vi "mxwScript_API_XMLMakeTargetRefText.vi"(6 "relativeToExistData":T1, 8 "templateData":T5={"tag"="", "index"=-1, "targetRefTemplateType"=enum."OutputAverage", "referencePosition"=enum."Right", "terminalData"={"name"="", "termIsTag"=FALSE, "referencePosition"=enum."TopLeft"}}, 9 "absoluteData":T4, 10 "terminalData":T3, 11 "targetRefType":T2) -> (3 "targetRefText":string)   [LabVIEW 2020]
uses:
  codeGenAPISupport.llb/cgAPI_mxwScript_DrpTmplt_TargetRefTemplateData.ctl
  codeGenAPISupport.llb/cgAPI_mxwScript_DrpTmplt_TargetRefTemplateType.ctl
  codeGenAPISupport.llb/cgAPI_mxwScript_DrpTmplt_ReferencePosition.ctl
  codeGenAPISupport.llb/cgAPI_mxwScript_DrpTmplt_TerminalData.ctl
  codeGenAPISupport.llb/cgAPI_mxwScript_DrpTmplt_AbsoluteData.ctl
  codeGenAPISupport.llb/cgAPI_mxwScript_DrpTmplt_TargetRefType.ctl
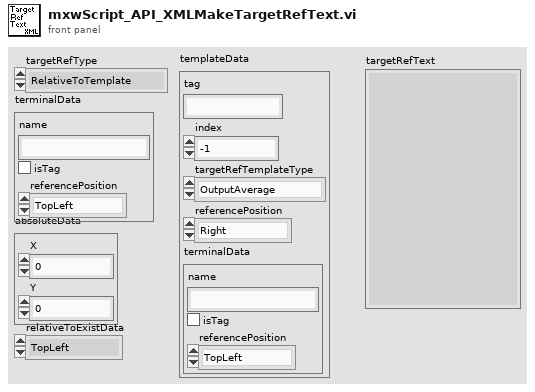
[diagram p1: front panel]
types:
  T1 = typedef "cgAPI_mxwScript_DrpTmplt_ReferencePosition.ctl" = enum16{"TopLeft", "Top", "TopRight", "Left", "Middle", "Right", "BottomLeft", "Bottom", "BottomRight"}
  T2 = typedef "cgAPI_mxwScript_DrpTmplt_TargetRefType.ctl" = enum16{"RelativeToTemplate", "RelativeToTerminal", "AbsoluteOnRoot", "AbsoluteOnTarget", "RelativeToExistOnRoot"}
  T3 = typedef "cgAPI_mxwScript_DrpTmplt_TerminalData.ctl" = cluster{"name":string, "termIsTag":bool, "referencePosition":T1}
  T4 = typedef "cgAPI_mxwScript_DrpTmplt_AbsoluteData.ctl" = cluster{"X":i32, "Y":i32}
  T5 = typedef "cgAPI_mxwScript_DrpTmplt_TargetRefTemplateData.ctl" = cluster{"tag":string, "index":i32, "targetRefTemplateType":T6, "referencePosition":T1, "terminalData":T3}
  T6 = typedef "cgAPI_mxwScript_DrpTmplt_TargetRefTemplateType.ctl" = enum16{"OutputAverage", "Absolute", "Terminal"}
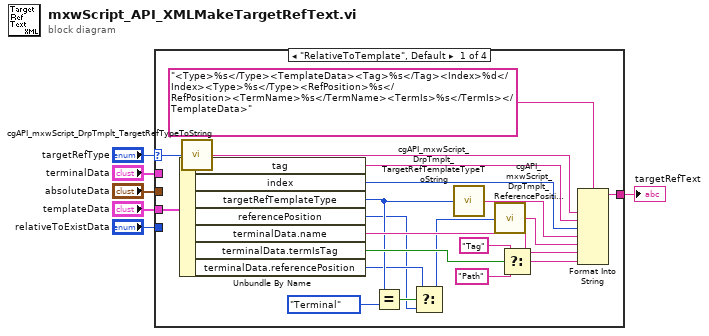
[diagram p0: block diagram]
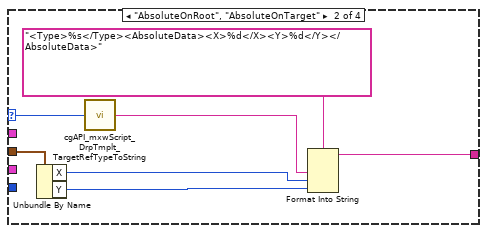
[diagram p2: hidden frame]
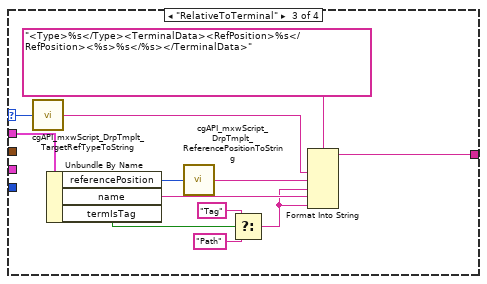
[diagram p3: hidden frame]
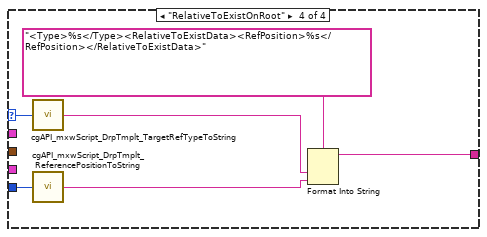
[diagram p4: hidden frame]
diagram:
  n1 = case shown="\"RelativeToTemplate\", Default" "targetRefType" {
    selector: "targetRefType" -> [w13 w28 w37 w49]
    tunnel: "terminalData" -> [_ _ w39 _]
    tunnel: "absoluteData" -> [_ w31 _ _]
    tunnel: "templateData" -> [w26 _ _ _]
    tunnel: [w15 w32 w40 w50] -> w6
    tunnel: "relativeToExistData" -> [_ _ _ w47]
    frame "RelativeToTemplate", Default {
      n2 = Unbundle By Name(w26) -> ("tag"=w24:string, "index"=w23:i32, "targetRefTemplateType"=w12:T6, "referencePosition"=w8:T1, "terminalData.name"=w20:string, "terminalData.termIsTag"=w19:bool, "terminalData.referencePosition"=w9:T1)
      n3 = call "cgAPI_mxwScript_DrpTmplt_TargetRefTypeToString.vi"("targetRefType"=w13) -> ("string"=w14:string)  [unwired: 4 out]
      n4 = Equal?(x=w12, y=cgAPI_mxwScript_DrpTmplt_TargetRefTemplateType."Terminal") -> (x = y?=w10:bool)
      n5 = Select(t=w9, s=w10, f=w8) -> (s? t:f=w7:T1)
      n6 = call "cgAPI_mxwScript_DrpTmplt_TargetRefTemplateTypeToString.vi"("targetRefTemplateType"=w12) -> ("string"=w22:string)  [unwired: 4 out]
      n7 = call "cgAPI_mxwScript_DrpTmplt_ReferencePositionToString.vi"("referencePosition"=w7) -> ("string"=w21:string)  [unwired: 4 out]
      n8 = Select(t="Tag", s=w19, f="Path") -> (s? t:f=w16:string)
      n9 = Format Into String(format string="<Type>%s</Type><TemplateData><Tag>%s</Tag><Index>%d</Index><Type>%s</Type><RefPosition>%s</RefPosition><TermName>%s</TermName><TermIs>%s</TermIs></TemplateData>", w14, w24, w23, w22, w21, w20, w16) -> (resulting string=w15:string)  [unwired: 2 in, 1 out]
    }
    frame "AbsoluteOnRoot", "AbsoluteOnTarget" {
      n10 = Unbundle By Name(w31) -> ("X"=w30:i32, "Y"=w29:i32)
      n11 = call "cgAPI_mxwScript_DrpTmplt_TargetRefTypeToString.vi"("targetRefType"=w28) -> ("string"=w27:string)  [unwired: 4 out]
      n12 = Format Into String(format string="<Type>%s</Type><AbsoluteData><X>%d</X><Y>%d</Y></AbsoluteData>", w27, w30, w29) -> (resulting string=w32:string)  [unwired: 2 in, 1 out]
    }
    frame "RelativeToTerminal" {
      n13 = call "cgAPI_mxwScript_DrpTmplt_TargetRefTypeToString.vi"("targetRefType"=w37) -> ("string"=w36:string)  [unwired: 4 out]
      n14 = Unbundle By Name(w39) -> ("referencePosition"=w35:T1, "name"=w44:string, "termIsTag"=w43:bool)
      n15 = call "cgAPI_mxwScript_DrpTmplt_ReferencePositionToString.vi"("referencePosition"=w35) -> ("string"=w34:string)  [unwired: 4 out]
      n16 = Select(t="Tag", s=w43, f="Path") -> (s? t:f=w38:string)
      n17 = Format Into String(format string="<Type>%s</Type><TerminalData><RefPosition>%s</RefPosition><%s>%s</%s></TerminalData>", w36, w34, w38, w44, w38) -> (resulting string=w40:string)  [unwired: 2 in, 1 out]
    }
    frame "RelativeToExistOnRoot" {
      n18 = call "cgAPI_mxwScript_DrpTmplt_TargetRefTypeToString.vi"("targetRefType"=w49) -> ("string"=w48:string)  [unwired: 4 out]
      n19 = call "cgAPI_mxwScript_DrpTmplt_ReferencePositionToString.vi"("referencePosition"=w47) -> ("string"=w46:string)  [unwired: 4 out]
      n20 = Format Into String(format string="<Type>%s</Type><RelativeToExistData><RefPosition>%s</RefPosition></RelativeToExistData>", w48, w46) -> (resulting string=w50:string)  [unwired: 2 in, 1 out]
    }
  }
  "targetRefText" <- w6
